vi "Read Method Information.vi"(8 "error in (no error)":errorcluster, 9 "Method":string, 10 "Function Block":string, 11 "TwinCAT ADS in":refnum<class "TwinCAT ADS.lvclass">) -> (0 "error out":errorcluster, 1 "Method Information":T1 {"Parameters"."Parameter Flags" items=["In"=1, "Out"=2, "ByReference"=4, "MaskIn"=5, "MaskOut"=6]}, 3 "TwinCAT ADS out":refnum<class "TwinCAT ADS.lvclass">)   [LabVIEW 2018, in "TwinCAT ADS.lvclass"]
uses:
  TwinCAT ADS.lvclass
  Controls/Method Information.ctl
  Controls/Method Parameter Information.ctl
  TwinCAT ADS.lvclass/TwinCAT ADS.ctl
  TwinCAT.Ads
  Get From Symbol Map.vi
  Get From Symbol Map Daemon.vi
  Get Symbol Map.vi
  Format String.vi
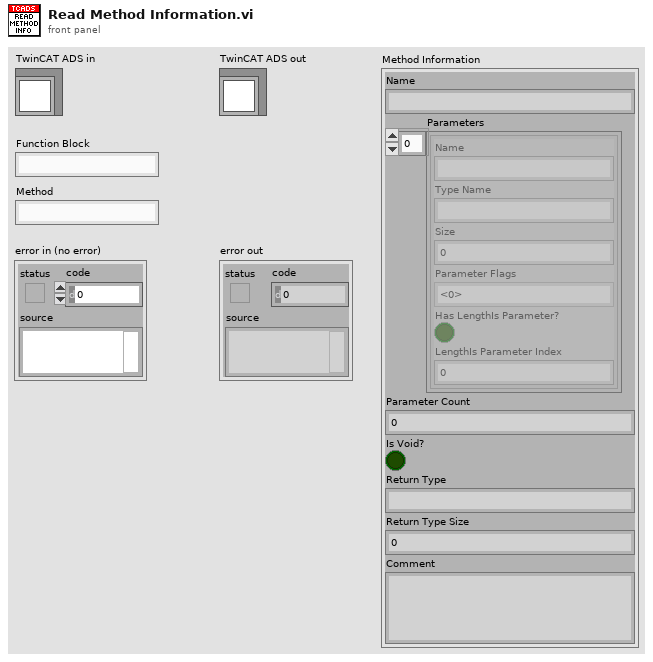
[diagram p1: front panel]
types:
  T1 = typedef "TwinCAT ADS.lvclass/Method Information.ctl" = cluster{"Name":string, "Parameters":T2[], "Parameter Count":i32, "Is Void?":bool, "Return Type":string, "Return Type Size":i32, "Comment":string}
  T2 = typedef "TwinCAT ADS.lvclass/Method Parameter Information.ctl" = cluster{"Name":string, "Type Name":string, "Size":i32, "Parameter Flags":u32, "Has LengthIs Parameter?":bool, "LengthIs Parameter Index":i32}
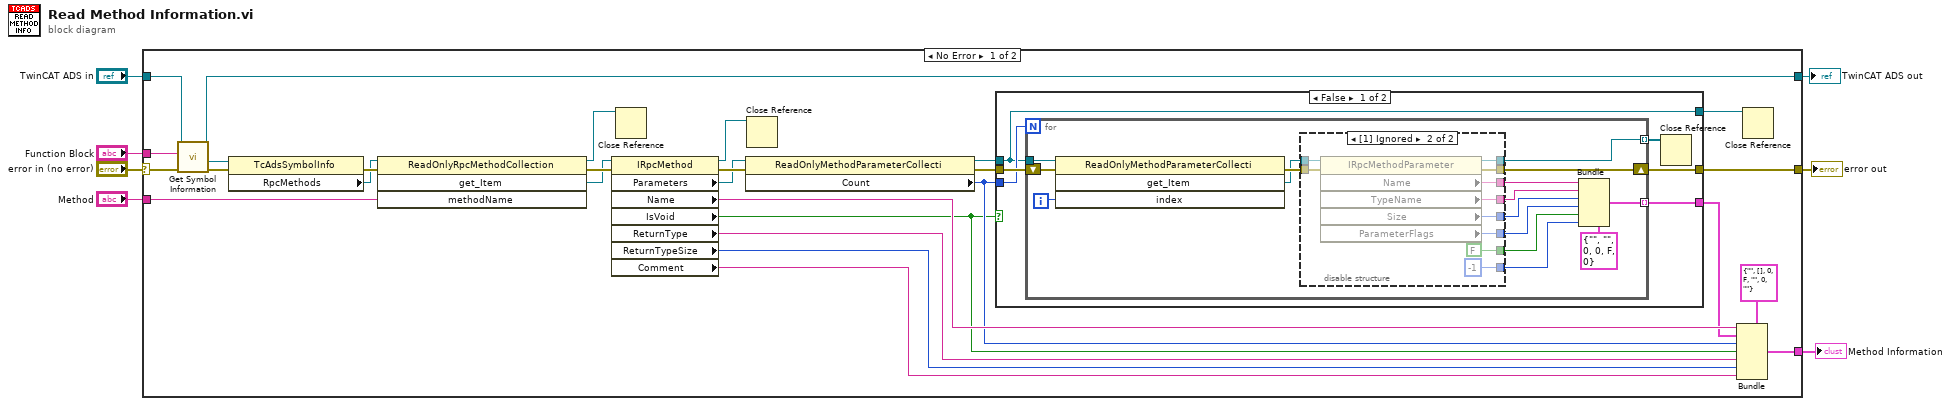
[diagram p0: block diagram]
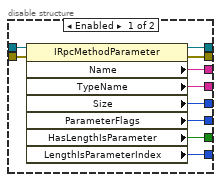
[diagram p2: hidden frame]
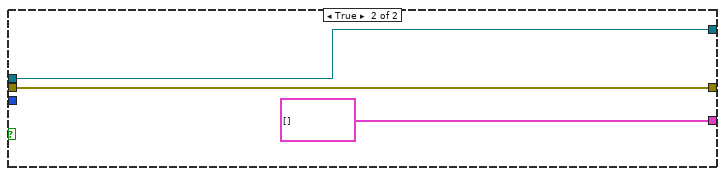
[diagram p3: hidden frame]
diagram:
  n1 = case shown="No Error" "error in (no error)" {
    selector: "error in (no error)" -> [w12 w81]
    tunnel: [w25 w81] -> w6
    tunnel: [w8 w80] -> w4
    tunnel: "TwinCAT ADS in" -> [w9 w80]
    tunnel: "Function Block" -> [w11 _]
    tunnel: "Method" -> [w33 _]
    tunnel: [w24 _] -> w1
    frame No Error {
      n2 = call "Get Symbol Information.vi"("error in (no error)"=w12, "Symbol Name"=w11, "TwinCAT ADS in"=w9) -> ("error out"=w13:errorcluster, ".NET Symbol Information"=w10:refnum<k24>, "TwinCAT ADS out"=w8:refnum<class "TwinCAT ADS.lvclass">)  [unwired: 6 in]
      n3 = property class="TcAdsSymbolInfo"(reference=w10, error in=w13) -> (error out=w34:errorcluster, "RpcMethods"=w18:refnum<k24>)  [unwired: 1 out]
      n4 = invoke class="ReadOnlyRpcMethodCollection" method="get_Item"(reference=w18, error in=w34, "methodName"=w33) -> (reference out=w16:refnum<k24>, error out=w32:errorcluster, "get_Item"=w17:refnum<k24>)  [unwired: 1 in, 1 out]
      n5 = property class="IRpcMethod"(reference=w17, error in=w32) -> (reference out=w15:refnum<k24>, error out=w31:errorcluster, "Parameters"=w30:refnum<k24>, "Name"=w28:string, "IsVoid"=w22:bool, "ReturnType"=w21:string, "ReturnTypeSize"=w20:i32, "Comment"=w19:string)
      n6 = Close Reference(reference=w16) -> ()  [unwired: 1 in, 1 out]
      n7 = property class="ReadOnlyMethodParameterCollecti"(reference=w30, error in=w31) -> (reference out=w29:refnum<k24>, error out=w35:errorcluster, "Count"=w23:i32)
      n8 = Close Reference(reference=w15) -> ()  [unwired: 1 in, 1 out]
      n9 = case shown="False" w22 {
        tunnel: w35 -> [w41 w78]
        tunnel: w23 -> [w40 _]
        tunnel: w29 -> [w37 w77]
        tunnel: [w39 T2[] []] -> w27
        tunnel: [w38 w78] -> w25
        tunnel: [w37 w77] -> w14
        frame False {
          n10 = for {
            N: w40 -> [_]
            tunnel: w37 -> [w55]
            shift-right: [w44] -> w38
            shift-left: w41 -> [w56]
            tunnel: [w45] -> w39 mode=indexing
            tunnel: [w42] -> w36 mode=indexing
            i -> [w54]
            n11 = invoke class="ReadOnlyMethodParameterCollecti" method="get_Item"(reference=w55, error in=w56, "index"=w54) -> (error out=w53:errorcluster, "get_Item"=w52:refnum<k24>)  [unwired: 1 in, 2 out]
            n12 = disable-structure shown="[1] Ignored" {
              disable-tunnel: w53 -> [w66 w76]
              disable-tunnel: w52 -> [w65 w75]
              disable-tunnel: [w64 w71] -> w51
              disable-tunnel: [w63 w72] -> w50
              disable-tunnel: [w62 w73] -> w49
              disable-tunnel: [w61 FALSE ("HasLengthIsParameter")] -> w48
              disable-tunnel: [w60 -1 ("LengthIsParameterIndex")] -> w47
              disable-tunnel: [w59 w74] -> w46
              disable-tunnel: [w58 w70] -> w44
              disable-tunnel: [w57 w69] -> w42
              frame Enabled {
                n13 = property class="IRpcMethodParameter"(reference=w65, error in=w66) -> (reference out=w57:refnum<k24>, error out=w58:errorcluster, "Name"=w64:string, "TypeName"=w63:string, "Size"=w62:i32, "ParameterFlags"=w59:u32, "HasLengthIsParameter"=w61:bool, "LengthIsParameterIndex"=w60:i32)
              }
              frame Disabled {
                n14 = property class="IRpcMethodParameter"(reference=w75, error in=w76) -> (reference out=w69:refnum<k24>, error out=w70:errorcluster, "Name"=w71:string, "TypeName"=w72:string, "Size"=w73:i32, "ParameterFlags"=w74:u32)
              }
            }
            n15 = Bundle(cluster=T2 {"Name"="", "Type Name"="", "Size"=0, "Parameter Flags"=0, "Has LengthIs Parameter?"=FALSE, "LengthIs Parameter Index"=0} ("Method Parameter Infomation"), "Name"=w51, "Type Name"=w50, "Size"=w49, "Parameter Flags"=w46, "Has LengthIs Parameter?"=w48, "LengthIs Parameter Index"=w47) -> (w45:T2)
          }
          n16 = Close Reference(reference=w36) -> ()  [unwired: 1 in, 1 out]
        }
        frame True {
        }
      }
      n17 = Bundle(cluster=T1 {"Name"="", "Parameters"=[], "Parameter Count"=0, "Is Void?"=FALSE, "Return Type"="", "Return Type Size"=0, "Comment"=""} ("Method Information"), "Name"=w28, "Parameters"=w27, "Parameter Count"=w23, "Is Void?"=w22, "Return Type"=w21, "Return Type Size"=w20, "Comment"=w19) -> (w24:T1)
      n18 = Close Reference(reference=w14) -> ()  [unwired: 1 in, 1 out]
    }
    frame Error {
    }
  }
  "error out" <- w6
  "TwinCAT ADS out" <- w4
  "Method Information" <- w1
